vi "Init Instruments.vi"(8 "Error In":errorcluster, 11 "reference in":refnum<class "Measure and Stimulus Subsystems.lvclass">) -> (0 "Error Out":errorcluster, 3 "reference out":refnum<class "Measure and Stimulus Subsystems.lvclass">)   [LabVIEW 2023]
uses:
  Measure and Stimulus Subsystems.lvclass
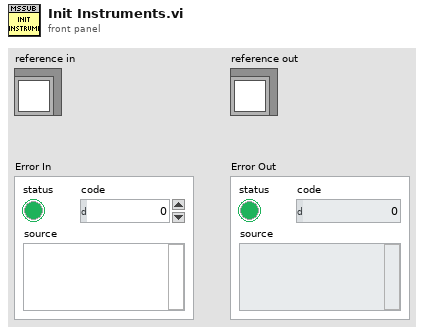
[diagram p1: front panel]
types:
  T1 = typedef "HAL GOOP4.lvlib/Measure and Stimulus Subsystems.lvclass/ObjectAttributes.ctl" = cluster{"Physical Instr":map{string, cluster{"IInstrument Base":refnum<class "IInstrument Base.lvclass">, "Initialized":bool}}, "Resource Mapping":map{string, cluster{"Instr Identifier":string, "Channel":u8}}}
  T2 = map{string, cluster{"IInstrument Base":refnum<class "IInstrument Base.lvclass">, "Initialized":bool}}
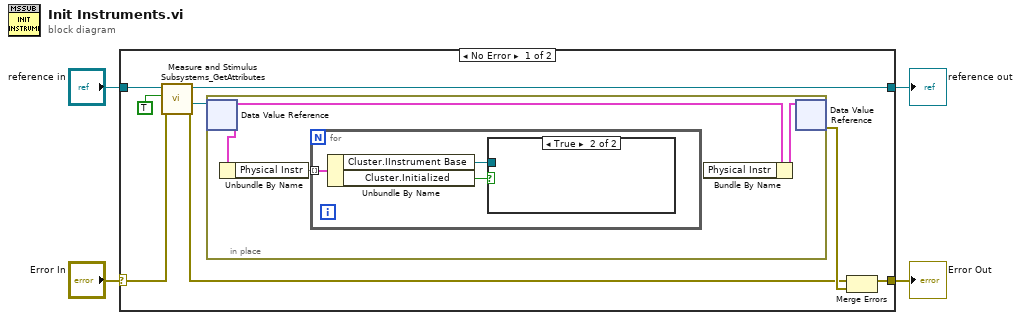
[diagram p0: block diagram]
diagram:
  n1 = case shown="No Error" "Error In" {
    selector: "Error In" -> [w11 w20]
    tunnel: [w8 w20] -> w3
    tunnel: [w9 w19] -> w1
    tunnel: "reference in" -> [w12 w19]
    frame No Error {
      n2 = call "Measure and Stimulus Subsystems_GetAttributes.vi"("Error In"=w11, "OnlyGetDvrReference(False)"=TRUE, "reference in"=w12) -> ("Error Out"=w6:errorcluster, "DataRef"=w7:refnum<data-value>, "reference out"=w9:refnum<class "Measure and Stimulus Subsystems.lvclass">)  [unwired: 5 in, 1 out]
      n3 = in-place {
        n4 = in-place-dvr #1(w7) -> (w14:T1)  [unwired: 1 out]
        n5 = Unbundle By Name(w14) -> ("Physical Instr"=w13:T2)
        n6 = for {
          tunnel: w13 -> [w18] mode=indexing
          n7 = Unbundle By Name(w18) -> ("Cluster.IInstrument Base"=w16:refnum<class "IInstrument Base.lvclass">, "Cluster.Initialized"=w17:bool)
          n8 = case shown="True" w17 {
            tunnel: w16 -> [_ _]
            frame False {
            }
            frame True {
            }
          }
        }
        n9 = Bundle By Name(cluster=w14) -> (w15:T1)  [unwired: 1 in]
        n10 = in-place-dvr #1(w15) -> (w10:errorcluster)  [unwired: 1 out]
      }
      n11 = Merge Errors(w6, w10) -> (w8:errorcluster)
    }
    frame Error {
    }
  }
  "Error Out" <- w3
  "reference out" <- w1
